vi "QDM_Main.vi"() -> ()   [LabVIEW 2020]
uses:
  <vilib>/userDefined/High Color/IMAQdx.ctl
panel:
  in  "Tab Control":T1(tab)
  in  "polarity pattern file":path
  in  "filename (adds .mat)":string="run_"
  in  "path":path
  in  "iterations":i32=1
  in  "SAVE":bool=TRUE
  in  "?":bool
  in  "Field (Gauss)":u16(ring)=1 items=["9G"=1, "14G"=2]
  out "num coil iters done":i32
  out "total pos sweeps":i32
  out "total neg sweeps":i32
  out "numSweeps list":i64[](array[numeric])=[10, 20, 10, 10, 20, 10]
  out "polarity list":i64[](array[numeric])=[-1, 1, -1, 1, -1, 1]
  out "coil polarity":bool=TRUE
  in  "freq range":T2(ring)=enum."Both ranges"
  out "num freqs\n(set by field)":i32(ring)=101 items=["51", "101"]
  in  "Height":i64(slide)=1200 min=0 max=1200 step=4 scale=0.0..1200.0
  in  "Width":i64(slide)=1920 min=0 max=1920 step=4 scale=0.0..1920.0
  in  "Arduino":refnum<visa-resource-name>="Arduino"
  in  "Helmholtz Coils":refnum<visa-resource-name>="BK9129B"
  in  "Camera Session In":T3="cam0"
  in  "TPI MW generator":refnum<visa-resource-name>="TPI"
  out "freq list (Hz)":dbl[](array[numeric])
  out "+Z current out (mA)":dbl=-975.0
  out "+Y current out (mA)":dbl=-1500.0
  out "+X current out (mA)":dbl=-20.0
  out "-Z current out (mA)":dbl=-975.0
  out "-Y current out (mA)":dbl=-1500.0
  out "-X current out (mA)":dbl=-20.0
  out "header cluster":T4
  out "img data stack pos":dbl[][](array[numeric])
  out "img data stack neg":dbl[][](array[numeric])
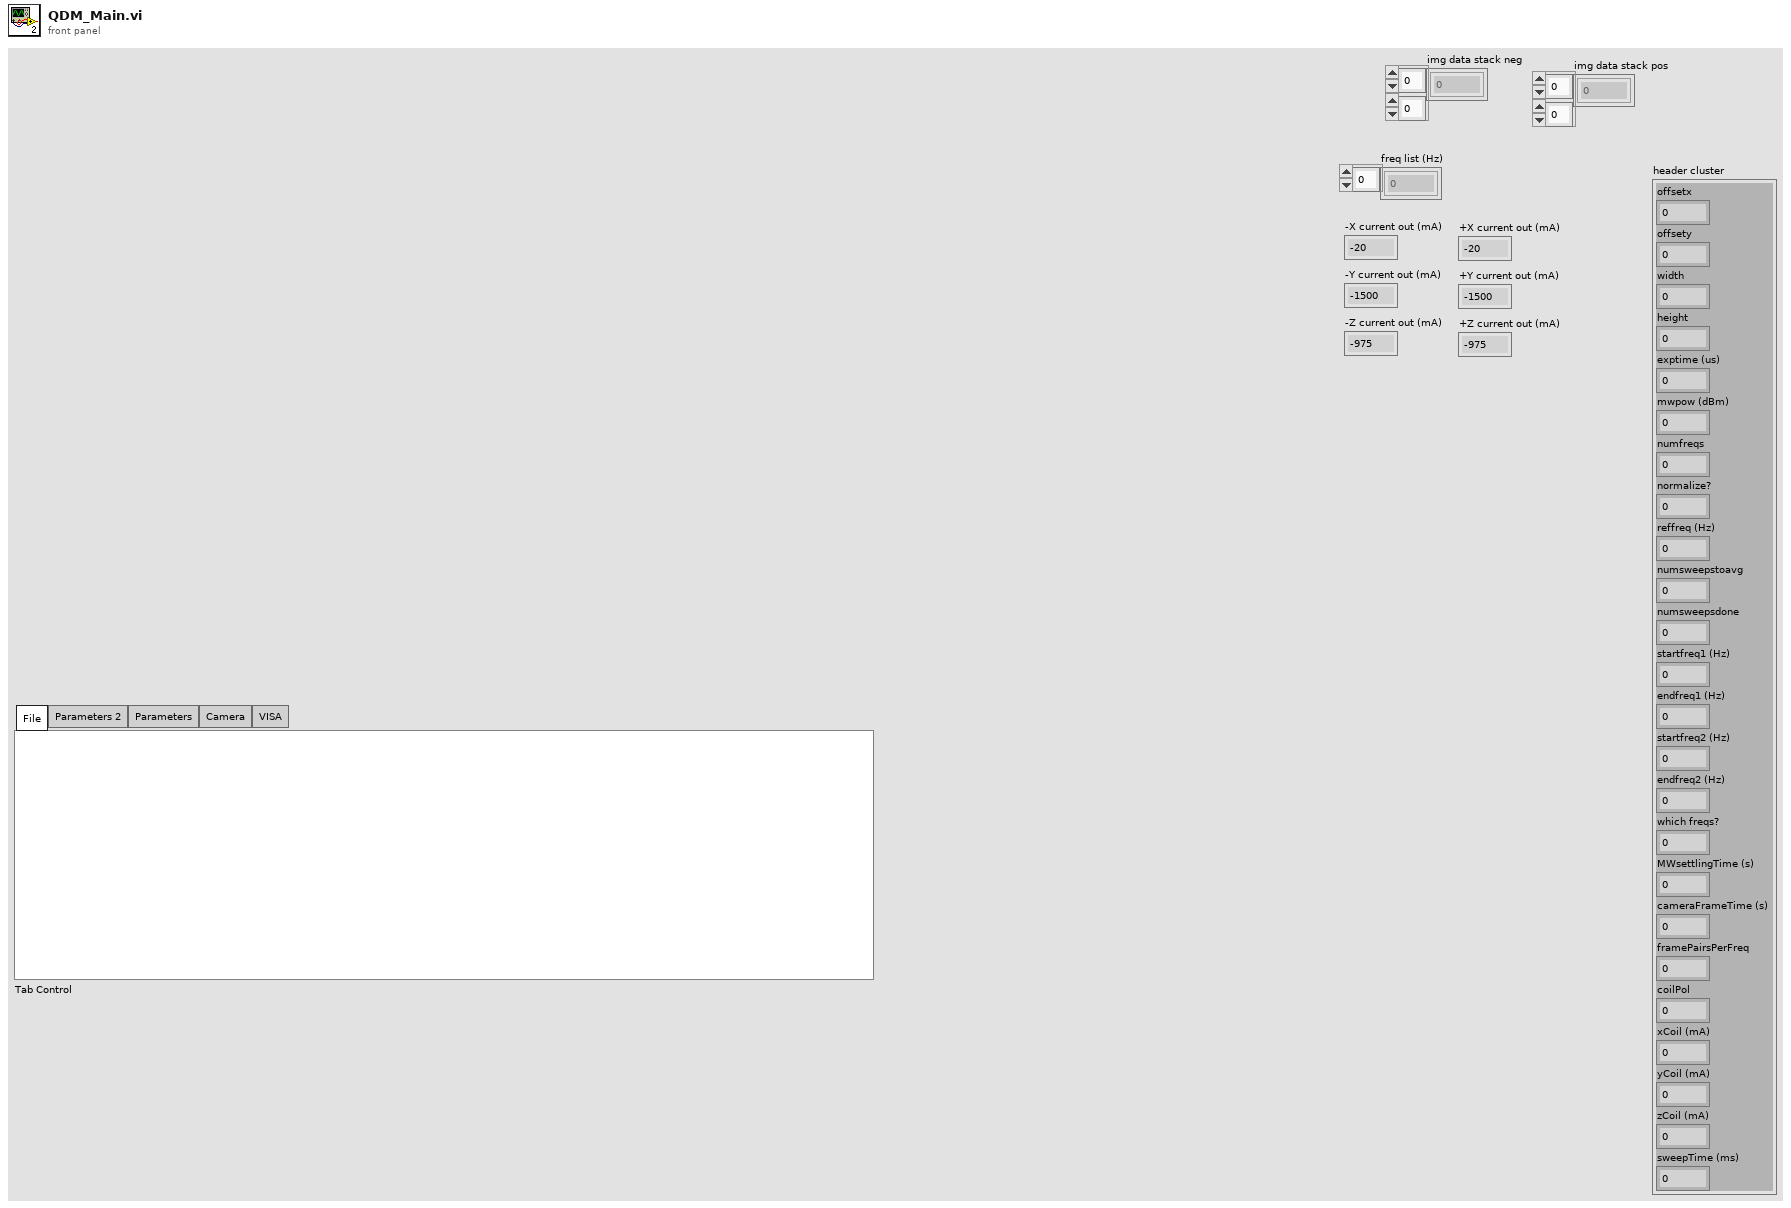
[diagram p1: front panel]
types:
  T1 = enum32{"File", "Parameters 2", "Parameters", "Camera", "VISA"}
  T2 = enum16{"Lower range", "Upper range", "Both ranges"}
  T3 = typedef "IMAQdx.ctl" = refnum<k21>
  T4 = cluster{"offsetx":i64, "offsety":i64, "width":i64, "height":i64, "exptime (us)":dbl, "mwpow (dBm)":dbl, "numfreqs":i32, "normalize?":i32, "reffreq (Hz)":dbl, "numsweepstoavg":i32, "numsweepsdone":i32, "startfreq1 (Hz)":dbl, "endfreq1 (Hz)":dbl, "startfreq2 (Hz)":dbl, "endfreq2 (Hz)":dbl, "which freqs?":i32, "MWsettlingTime (s)":dbl, "cameraFrameTime (s)":dbl, "framePairsPerFreq":i32, "coilPol":i32, "xCoil (mA)":dbl, "yCoil (mA)":dbl, "zCoil (mA)":dbl, "sweepTime (ms)":i32}
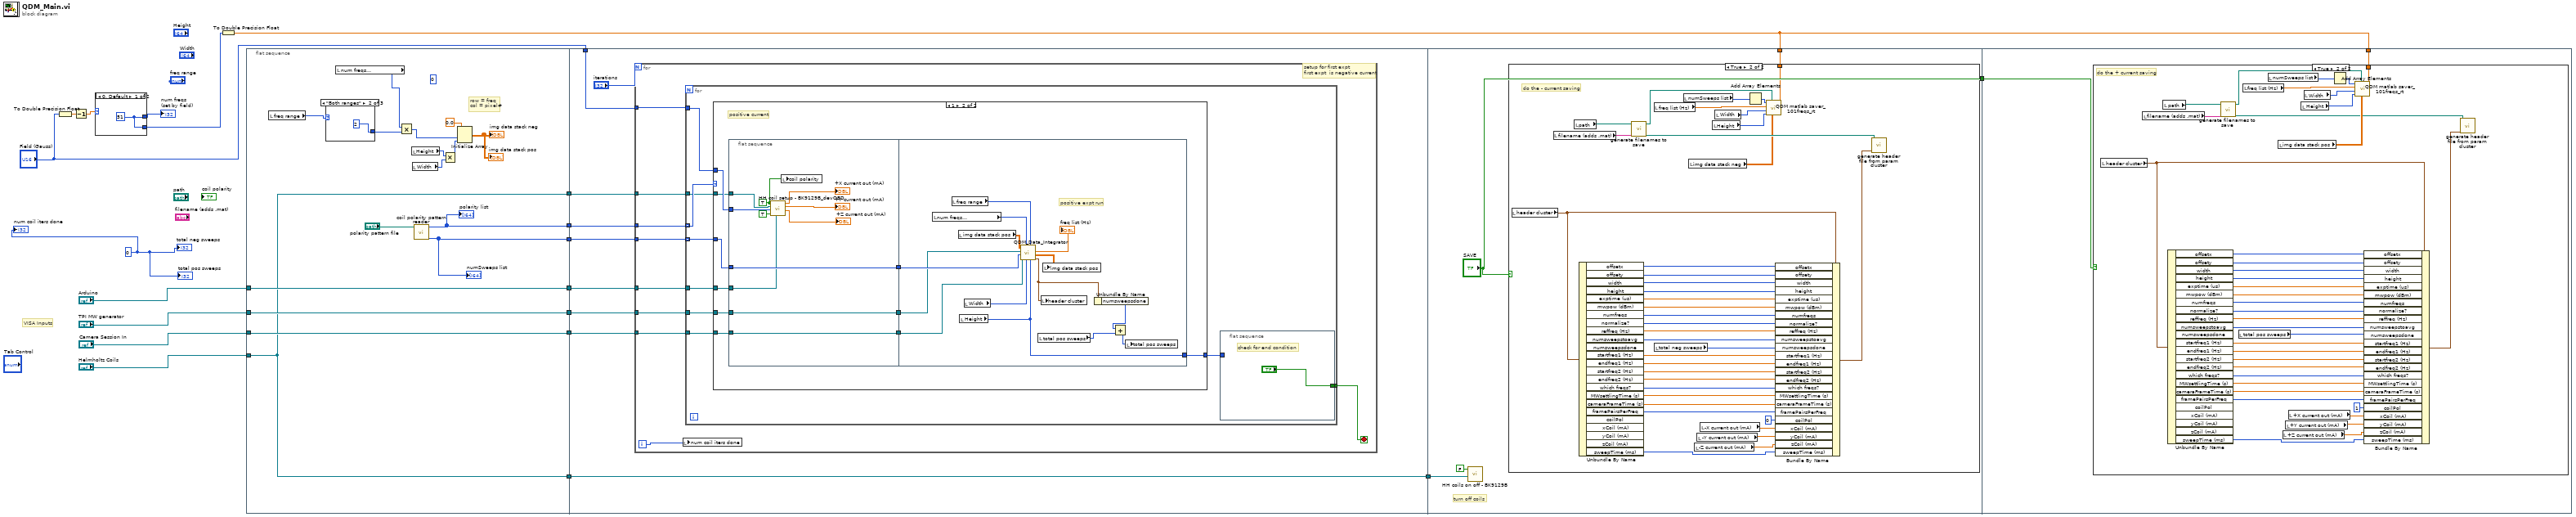
[diagram p0: block diagram]
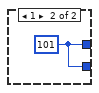
[diagram p2: hidden frame]
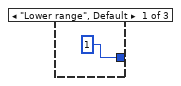
[diagram p3: hidden frame]
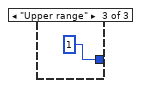
[diagram p4: hidden frame]
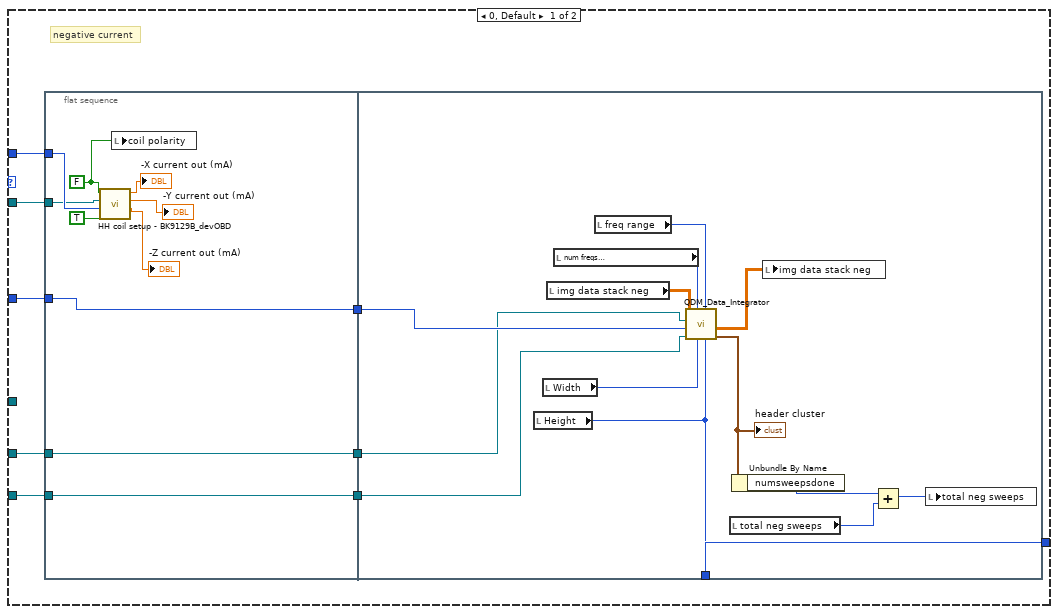
[diagram p5: hidden frame]
diagram:
  w18 = 0
  # "VISA Inputs"
  n1 = To Double Precision Float(number="Field (Gauss)") -> (double precision float=w14:dbl)
  n2 = Decrement(x=w14) -> (x-1=w13:dbl)
  n3 = case shown="0, Default" w13 {
    tunnel: [w21 w22] -> w15
    tunnel: [w21 w22] -> w12
    frame 0, Default {
      w21 = 51
    }
    frame 1 {
      w22 = 101
    }
  }
  "num freqs\n(set by field)" <- w15
  n4 = To Double Precision Float(number=w12) -> (double precision float=w11:dbl)
  n5 = flat-sequence {
    tunnel: [w28] -> w20
    tunnel: [w27] -> w19
    tunnel: [w24] -> w10
    tunnel: [w25] -> w9
    tunnel: [w23] -> w8
    tunnel: [w23] -> w6
    tunnel: [w26] -> w5
    tunnel: "Arduino" -> [w26]
    tunnel: "Camera Session In" -> [w25]
    tunnel: "TPI MW generator" -> [w24]
    tunnel: "Helmholtz Coils" -> [w23]
    tunnel: w20 -> [w50]
    tunnel: w19 -> [w49]
    tunnel: "Field (Gauss)" -> [w47]
    tunnel: w10 -> [w46]
    tunnel: w9 -> [w45]
    tunnel: w8 -> [w44]
    tunnel: [w43] -> w7
    tunnel: w6 -> [w43]
    tunnel: w5 -> [w42]
    tunnel: ["SAVE"] -> w17
    tunnel: w11 -> [w138]
    tunnel: w7 -> [w137]
    tunnel: w17 -> [w179]
    tunnel: w11 -> [w178]
    frame #0 {
      (unwired) 0 ("1st half sweeps")
      # "row = freq\ncol = pixel#"
      n6 = local read "freq range"() -> (w30:T2)
      n7 = case shown="\"Both ranges\"" w30 {
        tunnel: [1 ("numFreqs") 2 ("numFreqs") 1 ("numFreqs")] -> w33
        frame "Lower range", Default {
        }
        frame "Both ranges" {
        }
        frame "Upper range" {
        }
      }
      n8 = local read "num freqs\n(set by field)"() -> (w31:i32)
      n9 = Multiply(x=w31, y=w33) -> (x*y=w32:i32)
      n10 = local read "Height"() -> (w38:i64)
      n11 = local read "Width"() -> (w37:i64)
      n12 = call "coil polarity pattern reader.vi"("polarity pattern file"="polarity pattern file") -> ("numSweeps list"=w27:i64[], "polarity list"=w28:i64[])  [unwired: 9 in]
      "polarity list" <- w28
      "numSweeps list" <- w27
      n13 = Multiply(x=w38, y=w37) -> (x*y=w36:i64)
      n14 = Initialize Array(0.0 ("element"), w32, w36) -> (→"img data stack pos" →"img data stack neg":dbl[][])
    }
    frame #1 {
      n15 = for {
        N: "iterations" -> [_]
        tunnel: w50 -> [w59]
        tunnel: w49 -> [w58]
        tunnel: w47 -> [w55]
        tunnel: w46 -> [w54]
        tunnel: w45 -> [w53]
        tunnel: w44 -> [w52]
        tunnel: w42 -> [w51]
        i -> [w56]
        stop <- w57 stop-if-true
        # "setup for first expt\nfirst expt  is negative current"
        n16 = local write "num coil iters done"(w56) -> ()
        n17 = for {
          tunnel: w59 -> [w68] mode=indexing
          tunnel: w58 -> [w67] mode=indexing
          tunnel: [w65] -> w57
          tunnel: w55 -> [w64]
          tunnel: w54 -> [w63]
          tunnel: w53 -> [w62]
          tunnel: w52 -> [w61]
          tunnel: w51 -> [w60]
          n18 = case shown="1" w68 {
            tunnel: w67 -> [w77 w111]
            tunnel: [w76 w109] -> w66
            tunnel: w64 -> [w75 w108]
            tunnel: w63 -> [w73 w106]
            tunnel: w62 -> [w71 w104]
            tunnel: w61 -> [w70 w103]
            tunnel: w60 -> [_ w102]
            frame 0, Default {
              # "negative current"
              n19 = flat-sequence {
                tunnel: [w88] -> w78
                tunnel: w77 -> [w88]
                tunnel: w75 -> [w82]
                tunnel: [w81] -> w74
                tunnel: w73 -> [w81]
                tunnel: [w80] -> w72
                tunnel: w71 -> [w80]
                tunnel: w70 -> [w79]
                tunnel: w78 -> [w96]
                tunnel: [w95] -> w76
                tunnel: w74 -> [w90]
                tunnel: w72 -> [w89]
                frame #0 {
                  w87 = FALSE ("coil polarity")
                  n20 = call "HH coil setup - BK9129B_devOBD.VI"("setup enabled?"=TRUE, "number"=w82, "VISA resource name"=w79, "coil polarity"=w87) -> ("Z current out (mA)"=→"-Z current out (mA)":dbl, "Y current out (mA)"=→"-Y current out (mA)":dbl, "X current out (mA)"=→"-X current out (mA)":dbl)  [unwired: 5 in]
                  n21 = local write "coil polarity"(w87) -> ()
                }
                frame #1 {
                  n22 = local read "Height"() -> (w95:i64)
                  n23 = local read "Width"() -> (w99:i64)
                  n24 = local read "img data stack neg"() -> (w97:dbl[][])
                  n25 = local read "num freqs\n(set by field)"() -> (w101:i32)
                  n26 = local read "freq range"() -> (w100:T2)
                  n27 = call "QDM_Data_Integrator.vi"("Height"=w95, "which freqs?"=w100, "Width"=w99, "numFreqs"=w101, "Session In"=w89, "num sweeps to avg"=w96, "TPI VISA in"=w90, "img data stack Input"=w97) -> ("header cluster"=w94:T4, "img data stack Return"=w98:dbl[][])  [unwired: 2 out]
                  "header cluster" <- w94
                  n28 = local read "total neg sweeps"() -> (w92:i32)
                  n29 = Unbundle By Name(w94) -> ("numsweepsdone"=w93:i32)
                  n30 = local write "img data stack neg"(w98) -> ()
                  n31 = Add(x=w93, y=w92) -> (x+y=w91:i32)
                  n32 = local write "total neg sweeps"(w91) -> ()
                }
              }
            }
            frame 1 {
              # "positive current"
              n33 = flat-sequence {
                tunnel: w111 -> [w117]
                tunnel: [w117] -> w110
                tunnel: w108 -> [w116]
                tunnel: [w115] -> w107
                tunnel: w106 -> [w115]
                tunnel: [w114] -> w105
                tunnel: w104 -> [w114]
                tunnel: w103 -> [w113]
                tunnel: w102 -> [w112]
                tunnel: w110 -> [w130]
                tunnel: [w129] -> w109
                tunnel: w107 -> [w124]
                tunnel: w105 -> [w123]
                frame #0 {
                  w118 = TRUE ("coil polarity")
                  n34 = call "HH coil setup - BK9129B_devOBD.VI"("Arduino VISA in"=w112, "setup enabled?"=TRUE, "number"=w116, "VISA resource name"=w113, "coil polarity"=w118) -> ("Z current out (mA)"=→"+Z current out (mA)":dbl, "Y current out (mA)"=→"+Y current out (mA)":dbl, "X current out (mA)"=→"+X current out (mA)":dbl)  [unwired: 4 in]
                  n35 = local write "coil polarity"(w118) -> ()
                }
                frame #1 {
                  # "positive expt run"
                  n36 = local read "num freqs\n(set by field)"() -> (w136:i32)
                  n37 = local read "freq range"() -> (w135:T2)
                  n38 = local read "img data stack pos"() -> (w131:dbl[][])
                  n39 = local read "Height"() -> (w129:i64)
                  n40 = local read "Width"() -> (w134:i64)
                  n41 = call "QDM_Data_Integrator.vi"("Height"=w129, "which freqs?"=w135, "Width"=w134, "numFreqs"=w136, "Session In"=w123, "num sweeps to avg"=w130, "TPI VISA in"=w124, "img data stack Input"=w131) -> ("header cluster"=w128:T4, "img data stack Return"=w132:dbl[][], "freq list (Hz)"=→"freq list (Hz)":dbl[])  [unwired: 1 out]
                  n42 = local read "total pos sweeps"() -> (w126:i32)
                  n43 = local write "header cluster"(w128) -> ()
                  n44 = local write "img data stack pos"(w132) -> ()
                  n45 = Unbundle By Name(w128) -> ("numsweepsdone"=w127:i32)
                  n46 = Add(x=w127, y=w126) -> (x+y=w125:i32)
                  n47 = local write "total pos sweeps"(w125) -> ()
                }
              }
            }
          }
          n48 = flat-sequence {
            tunnel: w66 -> [_]
            tunnel: ["?"] -> w65
            frame #0 {
              # "check for end condition"
            }
          }
        }
      }
    }
    frame #2 {
      # "turn off coils"
      n49 = call "HH coils on off - BK9129B.VI"("BKcoil VISA"=w137, "coils on?"=FALSE) -> ()  [unwired: 10 in]
      n50 = case shown="True" "SAVE" {
        tunnel: w138 -> [_ w141]
        frame False {
        }
        frame True {
          # "do the - current saving"
          n51 = local read "header cluster"() -> (w152:T4)
          n52 = local read "filename (adds .mat)"() -> (w176:string)
          n53 = local read "path"() -> (w177:path)
          n54 = Unbundle By Name(w152) -> ("offsetx"=w153:i64, "offsety"=w154:i64, "width"=w155:i64, "height"=w156:i64, "exptime (us)"=w157:dbl, "mwpow (dBm)"=w158:dbl, "numfreqs"=w159:i32, "normalize?"=w160:i32, "reffreq (Hz)"=w161:dbl, "numsweepstoavg"=w162:i32, "startfreq1 (Hz)"=w163:dbl, "endfreq1 (Hz)"=w164:dbl, "startfreq2 (Hz)"=w165:dbl, "endfreq2 (Hz)"=w166:dbl, "which freqs?"=w167:i32, "MWsettlingTime (s)"=w168:dbl, "cameraFrameTime (s)"=w169:dbl, "framePairsPerFreq"=w170:i32, "sweepTime (ms)"=w171:i32)  [unwired: 5 out]
          n55 = call "generate filenames to save.vi"("filename (adds .mat)"=w176, "path"=w177) -> ("header path"=w175:path, "matlab path"=w150:path)  [unwired: 8 in]
          n56 = local read "freq list (Hz)"() -> (w146:dbl[])
          n57 = local read "total neg sweeps"() -> (w142:i32)
          n58 = local read "numSweeps list"() -> (w144:i64[])
          n59 = local read "img data stack neg"() -> (w147:dbl[][])
          n60 = local read "-Z current out (mA)"() -> (w174:dbl)
          n61 = local read "-Y current out (mA)"() -> (w173:dbl)
          n62 = local read "-X current out (mA)"() -> (w172:dbl)
          n63 = local read "Height"() -> (w148:i64)
          n64 = local read "Width"() -> (w149:i64)
          n65 = Add Array Elements(numeric array=w144) -> (sum=w143:i64)
          n66 = call "QDM matlab saver_101freqs_rt.vi"("NumofFreq"=w141, "img data stack Input"=w147, "matlab path"=w150, "Height"=w148, "Width"=w149, "freq list (Hz)"=w146, "sweep #"=w143) -> ()  [unwired: 5 in]
          n67 = Bundle By Name(cluster=w152, "offsetx"=w153, "offsety"=w154, "width"=w155, "height"=w156, "exptime (us)"=w157, "mwpow (dBm)"=w158, "numfreqs"=w159, "normalize?"=w160, "reffreq (Hz)"=w161, "numsweepstoavg"=w162, "numsweepsdone"=w142, "startfreq1 (Hz)"=w163, "endfreq1 (Hz)"=w164, "startfreq2 (Hz)"=w165, "endfreq2 (Hz)"=w166, "which freqs?"=w167, "MWsettlingTime (s)"=w168, "cameraFrameTime (s)"=w169, "framePairsPerFreq"=w170, "coilPol"=0, "xCoil (mA)"=w172, "yCoil (mA)"=w173, "zCoil (mA)"=w174, "sweepTime (ms)"=w171) -> (w151:T4)
          n68 = call "generate header file from param cluster.vi"("output cluster"=w151, "header path (full)"=w175) -> ()  [unwired: 10 in]
        }
      }
    }
    frame #3 {
      n69 = case shown="True" w179 {
        tunnel: w178 -> [_ w180]
        frame False {
        }
        frame True {
          # "do the + current saving"
          n70 = local read "header cluster"() -> (w210:T4)
          n71 = local read "filename (adds .mat)"() -> (w186:string)
          n72 = local read "path"() -> (w185:path)
          n73 = Unbundle By Name(w210) -> ("offsetx"=w209:i64, "offsety"=w208:i64, "width"=w207:i64, "height"=w206:i64, "exptime (us)"=w205:dbl, "mwpow (dBm)"=w204:dbl, "numfreqs"=w203:i32, "normalize?"=w202:i32, "reffreq (Hz)"=w201:dbl, "numsweepstoavg"=w200:i32, "startfreq1 (Hz)"=w199:dbl, "endfreq1 (Hz)"=w198:dbl, "startfreq2 (Hz)"=w197:dbl, "endfreq2 (Hz)"=w196:dbl, "which freqs?"=w195:i32, "MWsettlingTime (s)"=w194:dbl, "cameraFrameTime (s)"=w193:dbl, "framePairsPerFreq"=w192:i32, "sweepTime (ms)"=w191:i32)  [unwired: 5 out]
          n74 = call "generate filenames to save.vi"("filename (adds .mat)"=w186, "path"=w185) -> ("header path"=w187:path, "matlab path"=w212:path)  [unwired: 8 in]
          n75 = local read "total pos sweeps"() -> (w181:i32)
          n76 = local read "freq list (Hz)"() -> (w216:dbl[])
          n77 = local read "numSweeps list"() -> (w183:i64[])
          n78 = local read "img data stack pos"() -> (w215:dbl[][])
          n79 = local read "+Z current out (mA)"() -> (w188:dbl)
          n80 = local read "+Y current out (mA)"() -> (w189:dbl)
          n81 = local read "+X current out (mA)"() -> (w190:dbl)
          n82 = local read "Height"() -> (w214:i64)
          n83 = local read "Width"() -> (w213:i64)
          n84 = Add Array Elements(numeric array=w183) -> (sum=w182:i64)
          n85 = call "QDM matlab saver_101freqs_rt.vi"("NumofFreq"=w180, "img data stack Input"=w215, "matlab path"=w212, "Height"=w214, "Width"=w213, "freq list (Hz)"=w216, "sweep #"=w182) -> ()  [unwired: 5 in]
          n86 = Bundle By Name(cluster=w210, "offsetx"=w209, "offsety"=w208, "width"=w207, "height"=w206, "exptime (us)"=w205, "mwpow (dBm)"=w204, "numfreqs"=w203, "normalize?"=w202, "reffreq (Hz)"=w201, "numsweepstoavg"=w200, "numsweepsdone"=w181, "startfreq1 (Hz)"=w199, "endfreq1 (Hz)"=w198, "startfreq2 (Hz)"=w197, "endfreq2 (Hz)"=w196, "which freqs?"=w195, "MWsettlingTime (s)"=w194, "cameraFrameTime (s)"=w193, "framePairsPerFreq"=w192, "coilPol"=1, "xCoil (mA)"=w190, "yCoil (mA)"=w189, "zCoil (mA)"=w188, "sweepTime (ms)"=w191) -> (w211:T4)
          n87 = call "generate header file from param cluster.vi"("output cluster"=w211, "header path (full)"=w187) -> ()  [unwired: 10 in]
        }
      }
    }
  }
  "total neg sweeps" <- w18
  "total pos sweeps" <- w18
  "num coil iters done" <- w18
